vi "Periodic Tasks.vi"(8 "error in":errorcluster) -> ()   [LabVIEW 2018]
doc: "This VI runs in parallel to other robot code. It can contain as many user-defined periodic loops as you need. These can carry out PID or other sorts of timed response."
uses:
  <vilib>/Rock Robotics/WPI/Utilities/WPI_GetSetVariantRefNum.vi
  Robot Global Data.vi
panel:
  out "Cargo Stop Current":dbl=10.0 format="%#_13g"
  out "Stop the grabber":bool
  out "Solenoid Voltage":dbl
  out "Input Voltage":dbl
  out "Compressor current (A)":dbl
  out "all currents (A)":dbl[](array[numeric]) caption="0\n1\n2\n3\n4\n5\n6\n7\n8\n9\n10\n11\n12\n13\n14\n15"
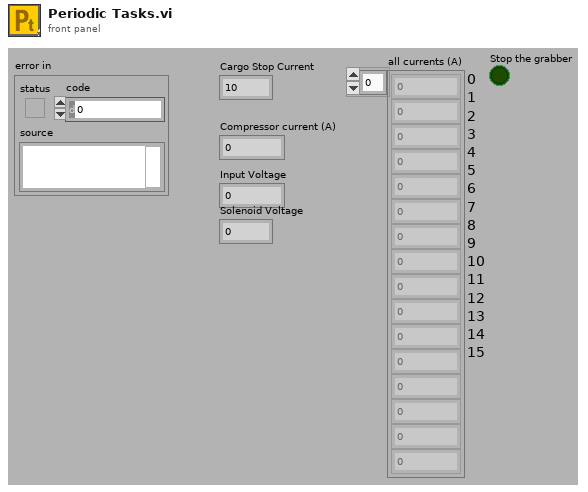
[diagram p1: front panel]
types:
  T1 = typedef "WPI_JoystickDevRef.ctl" = cluster{"Device":T2}
  T2 = typedef "WPI_JoystickDeviceEnum.ctl" = enum16{"USB 0", "USB 1", "USB 2", "USB 3", "USB 4", "USB 5"}
  T3 = cluster{"JoystickDevRef":T1, "JoystickDevRef":T1}
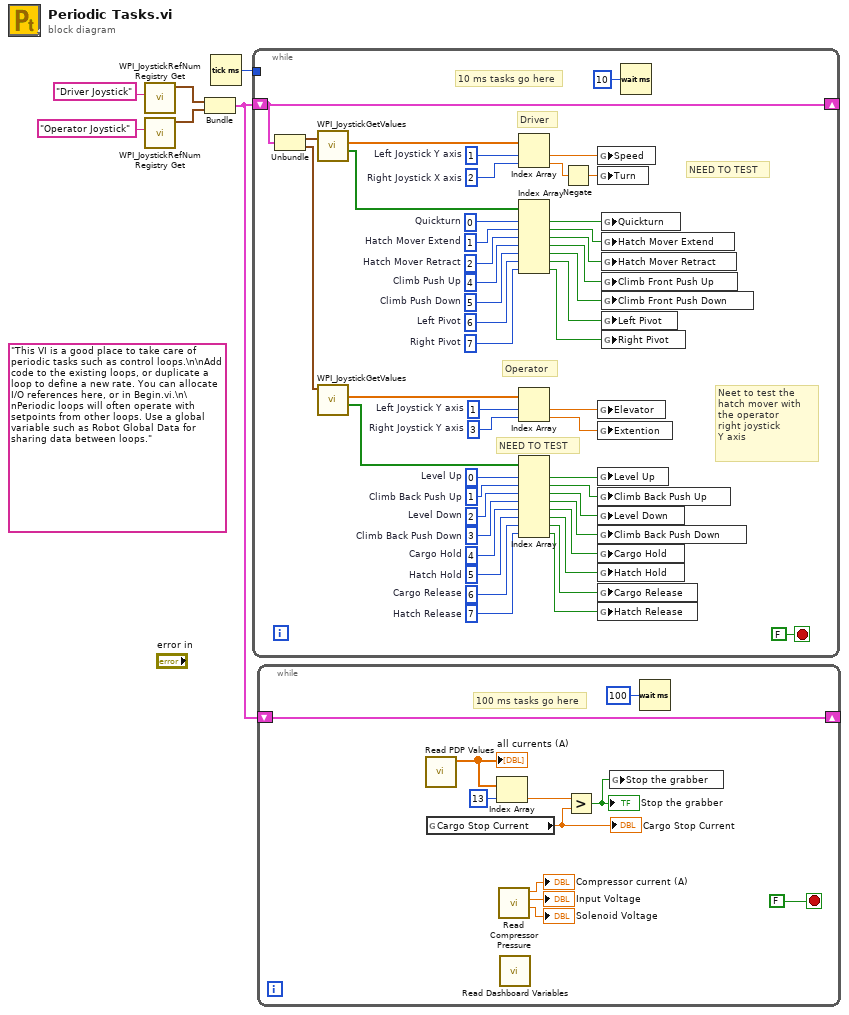
[diagram p0: block diagram]
diagram:
  (unwired) "This VI is a good place to take care of periodic tasks such as control loops.\n\nAdd code to the existing loops, or duplicate a loop to define a new rate. You can allocate I/O references here, or in Begin.vi.\n\nPeriodic loops will often operate with setpoints from other loops. Use a global variable such as Robot Global Data for sharing data between loops."
  n1 = call <vilib>:"WPI_JoystickRefNum Registry Get.vi"("refnum name"="Driver Joystick") -> ("JoystickDevRef"=w3:T1)  [unwired: 1 in, 9 out]
  n2 = call <vilib>:"WPI_JoystickRefNum Registry Get.vi"("refnum name"="Operator Joystick") -> ("JoystickDevRef"=w1:T1)  [unwired: 1 in, 9 out]
  n3 = Bundle("JoystickDevRef"=w3, "JoystickDevRef"=w1) -> (w2:T3)  [unwired: 1 in]
  n4 = Tick Count (ms)() -> (millisecond timer value=w5:u32)
  n5 = while {
    shift-right: [w49] -> _
    shift-left: w2 -> [w49]
    tunnel: w5 -> [_]
    stop <- FALSE stop-if-true
    w7 = 7  # Hatch Release
    w8 = 6  # Cargo Release
    w12 = 3  # Right Joystick Y axis
    w16 = 7  # Right Pivot
    w15 = 6  # Left Pivot
    w22 = 5  # Climb Push Down
    w23 = 4  # Climb Push Up
    w30 = 5  # Hatch Hold
    w31 = 4  # Cargo Hold
    w32 = 3  # Climb Back Push Down
    w33 = 2  # Level Down
    w34 = 1  # Climb Back Push Up
    w35 = 0  # Level Up
    w37 = 1  # Left Joystick Y axis
    w38 = 2  # Hatch Mover Retract
    w39 = 1  # Hatch Mover Extend
    w40 = 0  # Quickturn
    w43 = 2  # Right Joystick X axis
    w44 = 1  # Left Joystick Y axis
    # "10 ms tasks go here"
    # "Neet to test the\nhatch mover with\nthe operator \nright joystick\nY axis"
    # "Operator"
    # "Driver"
    # "NEED TO TEST"
    # "NEED TO TEST"
    n6 = Unbundle(w49) -> ("JoystickDevRef"=w48:T1, "JoystickDevRef"=w45:T1)
    n7 = call <vilib>:"WPI_JoystickGetValues.vi"("JoystickDevRef"=w48) -> ("Buttons"=w50:bool[], "Axes"=w52:dbl[])  [unwired: 6 in, 3 out]
    n8 = call <vilib>:"WPI_JoystickGetValues.vi"("JoystickDevRef"=w45) -> ("Buttons"=w47:bool[], "Axes"=w46:dbl[])  [unwired: 6 in, 3 out]
    n9 = Index Array(array=w52, index #1=w44, index #2=w43) -> (element #1=w42:dbl, element #2=w41:dbl)
    n10 = Index Array(array=w50, index #1=w40, index #2=w39, index #3=w38, index #4=w23, index #5=w22, index #6=w15, index #7=w16) -> (element #1=w21:bool, element #2=w20:bool, element #3=w19:bool, element #4=w18:bool, element #5=w17:bool, element #6=w13:bool, element #7=w14:bool)
    n11 = Index Array(array=w46, index #1=w37, index #2=w12) -> (element #1=w36:dbl, element #2=w11:dbl)
    n12 = Index Array(array=w47, index #1=w35, index #2=w34, index #3=w33, index #4=w32, index #5=w31, index #6=w30, index #7=w8, index #8=w7) -> (element #1=w29:bool, element #2=w28:bool, element #3=w27:bool, element #4=w26:bool, element #5=w25:bool, element #6=w24:bool, element #7=w10:bool, element #8=w9:bool)
    n13 = Negate(x=w41) -> (-x=w51:dbl)
    n14 = global write "Robot Global Data.vi" "Speed"(w42) -> ()
    n15 = global write "Robot Global Data.vi" "Turn"(w51) -> ()
    n16 = global write "Robot Global Data.vi" "Elevator"(w36) -> ()
    n17 = global write "Robot Global Data.vi" "Extention"(w11) -> ()
    n18 = global write "Robot Global Data.vi" "Level Up"(w29) -> ()
    n19 = global write "Robot Global Data.vi" "Climb Back Push Up"(w28) -> ()
    n20 = global write "Robot Global Data.vi" "Level Down"(w27) -> ()
    n21 = global write "Robot Global Data.vi" "Climb Back Push Down"(w26) -> ()
    n22 = global write "Robot Global Data.vi" "Cargo Hold"(w25) -> ()
    n23 = global write "Robot Global Data.vi" "Hatch Hold"(w24) -> ()
    n24 = global write "Robot Global Data.vi" "Cargo Release"(w10) -> ()
    n25 = global write "Robot Global Data.vi" "Hatch Release"(w9) -> ()
    n26 = global write "Robot Global Data.vi" "Quickturn"(w21) -> ()
    n27 = global write "Robot Global Data.vi" "Hatch Mover Extend"(w20) -> ()
    n28 = global write "Robot Global Data.vi" "Hatch Mover Retract"(w19) -> ()
    n29 = global write "Robot Global Data.vi" "Climb Front Push Up"(w18) -> ()
    n30 = global write "Robot Global Data.vi" "Climb Front Push Down"(w17) -> ()
    n31 = global write "Robot Global Data.vi" "Left Pivot"(w13) -> ()
    n32 = global write "Robot Global Data.vi" "Right Pivot"(w14) -> ()
    n33 = Wait (ms)(milliseconds to wait=u32 10) -> ()  [unwired: 1 out]
  }
  n34 = while {
    shift-right: [w63] -> _
    shift-left: w2 -> [w63]
    stop <- FALSE stop-if-true
    # "100 ms tasks go here"
    n35 = call "Read PDP Values.vi"() -> ("all currents (A)"=w57:dbl[])  [unwired: 11 in]
    "all currents (A)" <- w57
    n36 = global read "Robot Global Data.vi" "Cargo Stop Current"() -> (w59:dbl)
    "Cargo Stop Current" <- w59
    n37 = Index Array(array=w57, index=13) -> (element=w56:dbl)
    n38 = call "Read Compressor Pressure.vi"() -> ("Solenoid Voltage"=→"Solenoid Voltage":dbl, "Input Voltage"=→"Input Voltage":dbl, "Compressor current (A)"=→"Compressor current (A)":dbl)  [unwired: 9 in]
    n39 = call "Read Dashboard Variables.vi"() -> ()  [unwired: 12 in]
    n40 = Greater?(x=w56, y=w59) -> (0:w58:bool)
    "Stop the grabber" <- w58
    n41 = global write "Robot Global Data.vi" "Stop the grabber"(w58) -> ()
    n42 = Wait (ms)(milliseconds to wait=u32 100) -> ()  [unwired: 1 out]
  }
